vi "6_4.vi"() -> ()   [LabVIEW 2026]
panel:
  out "String":string
  out "moment of TRUTH":string
  out "index of \"n\"":dbl
  in  "\"n\"":dbl
  out "array o/p":dbl[](array[numeric])
  in  "read num-1D":dbl[](array[numeric])
  # "Create a VI to read a set of numbers and store it on the one-dimensional array and \nagain read a number ‘n’, and check whether it is present in the array. If it is so, print \nout the position of ‘n’ in the array and also check whether it repeats in the array"
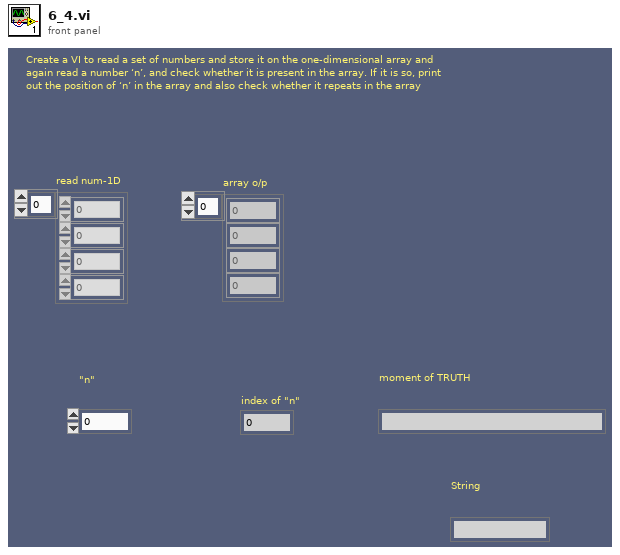
[diagram p1: front panel]
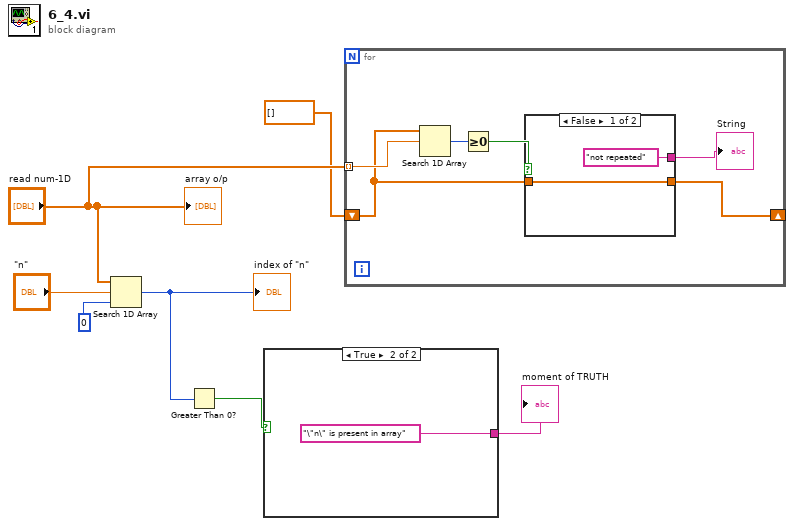
[diagram p0: block diagram]
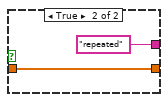
[diagram p2: hidden frame]
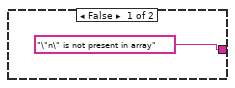
[diagram p3: hidden frame]
diagram:
  n1 = Search 1D Array(1D array="read num-1D", element="\"n\"", start index (0)=0) -> (index of element=w5:i32)
  "index of \"n\"" <- w5
  n2 = Greater Than 0?(x=w5) -> (x > 0?=w4:bool)
  n3 = case shown="True" w4 {
    tunnel: ["\"n\" is not present in array" "\"n\" is present in array"] -> w3
    frame False {
    }
    frame True {
    }
  }
  "moment of TRUTH" <- w3
  n4 = for {
    tunnel: "read num-1D" -> [w15] mode=indexing
    shift-right: [w11] -> _
    shift-left: dbl[] [] -> [w12]
    n5 = Search 1D Array(1D array=w12, element=w15) -> (index of element=w14:i32)  [unwired: 1 in]
    n6 = Greater Or Equal To 0?(x=w14) -> (x >= 0?=w13:bool)
    n7 = case shown="False" w13 {
      tunnel: [w17 w19] -> w11
      tunnel: w12 -> [w17 w19]
      tunnel: ["not repeated" "repeated"] -> w10
      frame False {
      }
      frame True {
      }
    }
    "String" <- w10
  }
  "array o/p" <- "read num-1D"
